vi "FipsAdjacent.vi"() -> (11 "Fips":i32[](array[numeric]))   [LabVIEW 2017] (continued)
\"Grand County, UT\"\t49019\n\"San Juan County, UT\"\t49037\t\"Kane County, UT\"\t49025\n\"San Juan County, UT\"\t49037\t\"San Juan County, UT\"\t49037\n\"San Juan County, UT\"\t49037\t\"Wayne County, UT\"\t49055\n\"Sanpete County, UT\"\t49039\t\"Carbon County, UT\"\t49007\n\"Sanpete County, UT\"\t49039\t\"Emery County, UT\"\t49015\n\"Sanpete County, UT\"\t49039\t\"Juab County, UT\"\t49023\n\"Sanpete County, UT\"\t49039\t\"Millard County, UT\"\t49027\n\"Sanpete County, UT\"\t49039\t\"Sanpete County, UT\"\t49039\n\"Sanpete County, UT\"\t49039\t\"Sevier County, UT\"\t49041\n\"Sanpete County, UT\"\t49039\t\"Utah County, UT\"\t49049\n\"Sevier County, UT\"\t49041\t\"Beaver County, UT\"\t49001\n\"Sevier County, UT\"\t49041\t\"Emery County, UT\"\t49015\n\"Sevier County, UT\"\t49041\t\"Millard County, UT\"\t49027\n\"Sevier County, UT\"\t49041\t\"Piute County, UT\"\t49031\n\"Sevier County, UT\"\t49041\t\"Sanpete County, UT\"\t49039\n\"Sevier County, UT\"\t49041\t\"Sevier County, UT\"\t49041\n\"Sevier County, UT\"\t49041\t\"Wayne County, UT\"\t49055\n\"Summit County, UT\"\t49043\t\"Daggett County, UT\"\t49009\n\"Summit County, UT\"\t49043\t\"Duchesne County, UT\"\t49013\n\"Summit County, UT\"\t49043\t\"Morgan County, UT\"\t49029\n\"Summit County, UT\"\t49043\t\"Rich County, UT\"\t49033\n\"Summit County, UT\"\t49043\t\"Salt Lake County, UT\"\t49035\n\"Summit County, UT\"\t49043\t\"Summit County, UT\"\t49043\n\"Summit County, UT\"\t49043\t\"Wasatch County, UT\"\t49051\n\"Summit County, UT\"\t49043\t\"Sweetwater County, WY\"\t56037\n\"Summit County, UT\"\t49043\t\"Uinta County, WY\"\t56041\n\"Tooele County, UT\"\t49045\t\"Elko County, NV\"\t32007\n\"Tooele County, UT\"\t49045\t\"White Pine County, NV\"\t32033\n\"Tooele County, UT\"\t49045\t\"Box Elder County, UT\"\t49003\n\"Tooele County, UT\"\t49045\t\"Davis County, UT\"\t49011\n\"Tooele County, UT\"\t49045\t\"Juab County, UT\"\t49023\n\"Tooele County, UT\"\t49045\t\"Salt Lake County, UT\"\t49035\n\"Tooele County, UT\"\t49045\t\"Tooele County, UT\"\t49045\n\"Tooele County, UT\"\t49045\t\"Utah County, UT\"\t49049\n\"Tooele County, UT\"\t49045\t\"Weber County, UT\"\t49057\n\"Uintah County, UT\"\t49047\t\"Garfield County, CO\"\t08045\n\"Uintah County, UT\"\t49047\t\"Moffat County, CO\"\t08081\n\"Uintah County, UT\"\t49047\t\"Rio Blanco County, CO\"\t08103\n\"Uintah County, UT\"\t49047\t\"Carbon County, UT\"\t49007\n\"Uintah County, UT\"\t49047\t\"Daggett County, UT\"\t49009\n\"Uintah County, UT\"\t49047\t\"Duchesne County, UT\"\t49013\n\"Uintah County, UT\"\t49047\t\"Emery County, UT\"\t49015\n\"Uintah County, UT\"\t49047\t\"Grand County, UT\"\t49019\n\"Uintah County, UT\"\t49047\t\"Uintah County, UT\"\t49047\n\"Utah County, UT\"\t49049\t\"Carbon County, UT\"\t49007\n\"Utah County, UT\"\t49049\t\"Duchesne County, UT\"\t49013\n\"Utah County, UT\"\t49049\t\"Juab County, UT\"\t49023\n\"Utah County, UT\"\t49049\t\"Salt Lake County, UT\"\t49035\n\"Utah County, UT\"\t49049\t\"Sanpete County, UT\"\t49039\n\"Utah County, UT\"\t49049\t\"Tooele County, UT\"\t49045\n\"Utah County, UT\"\t49049\t\"Utah County, UT\"\t49049\n\"Utah County, UT\"\t49049\t\"Wasatch County, UT\"\t49051\n\"Wasatch County, UT\"\t49051\t\"Duchesne County, UT\"\t49013\n\"Wasatch County, UT\"\t49051\t\"Salt Lake County, UT\"\t49035\n\"Wasatch County, UT\"\t49051\t\"Summit County, UT\"\t49043\n\"Wasatch County, UT\"\t49051\t\"Utah County, UT\"\t49049\n\"Wasatch County, UT\"\t49051\t\"Wasatch County, UT\"\t49051\n\"Washington County, UT\"\t49053\t\"Mohave County, AZ\"\t04015\n\"Washington County, UT\"\t49053\t\"Lincoln County, NV\"\t32017\n\"Washington County, UT\"\t49053\t\"Iron County, UT\"\t49021\n\"Washington County, UT\"\t49053\t\"Kane County, UT\"\t49025\n\"Washington County, UT\"\t49053\t\"Washington County, UT\"\t49053\n\"Wayne County, UT\"\t49055\t\"Emery County, UT\"\t49015\n\"Wayne County, UT\"\t49055\t\"Garfield County, UT\"\t49017\n\"Wayne County, UT\"\t49055\t\"Grand County, UT\"\t49019\n\"Wayne County, UT\"\t49055\t\"Piute County, UT\"\t49031\n\"Wayne County, UT\"\t49055\t\"San Juan County, UT\"\t49037\n\"Wayne County, UT\"\t49055\t\"Sevier County, UT\"\t49041\n\"Wayne County, UT\"\t49055\t\"Wayne County, UT\"\t49055\n\"Weber County, UT\"\t49057\t\"Box Elder County, UT\"\t49003\n\"Weber County, UT\"\t49057\t\"Cache County, UT\"\t49005\n\"Weber County, UT\"\t49057\t\"Davis County, UT\"\t49011\n\"Weber County, UT\"\t49057\t\"Morgan County, UT\"\t49029\n\"Weber County, UT\"\t49057\t\"Rich County, UT\"\t49033\n\"Weber County, UT\"\t49057\t\"Tooele County, UT\"\t49045\n\"Weber County, UT\"\t49057\t\"Weber County, UT\"\t49057\n\"Addison County, VT\"\t50001\t\"Essex County, NY\"\t36031\n\"Addison County, VT\"\t50001\t\"Washington County, NY\"\t36115\n\"Addison County, VT\"\t50001\t\"Addison County, VT\"\t50001\n\"Addison County, VT\"\t50001\t\"Chittenden County, VT\"\t50007\n\"Addison County, VT\"\t50001\t\"Orange County, VT\"\t50017\n\"Addison County, VT\"\t50001\t\"Rutland County, VT\"\t50021\n\"Addison County, VT\"\t50001\t\"Washington County, VT\"\t50023\n\"Addison County, VT\"\t50001\t\"Windsor County, VT\"\t50027\n\"Bennington County, VT\"\t50003\t\"Berkshire County, MA\"\t25003\n\"Bennington County, VT\"\t50003\t\"Franklin County, MA\"\t25011\n\"Bennington County, VT\"\t50003\t\"Rensselaer County, NY\"\t36083\n\"Bennington County, VT\"\t50003\t\"Washington County, NY\"\t36115\n\"Bennington County, VT\"\t50003\t\"Bennington County, VT\"\t50003\n\"Bennington County, VT\"\t50003\t\"Rutland County, VT\"\t50021\n\"Bennington County, VT\"\t50003\t\"Windham County, VT\"\t50025\n\"Bennington County, VT\"\t50003\t\"Windsor County, VT\"\t50027\n\"Caledonia County, VT\"\t50005\t\"Grafton County, NH\"\t33009\n\"Caledonia County, VT\"\t50005\t\"Caledonia County, VT\"\t50005\n\"Caledonia County, VT\"\t50005\t\"Essex County, VT\"\t50009\n\"Caledonia County, VT\"\t50005\t\"Lamoille County, VT\"\t50015\n\"Caledonia County, VT\"\t50005\t\"Orange County, VT\"\t50017\n\"Caledonia County, VT\"\t50005\t\"Orleans County, VT\"\t50019\n\"Caledonia County, VT\"\t50005\t\"Washington County, VT\"\t50023\n\"Chittenden County, VT\"\t50007\t\"Clinton County, NY\"\t36019\n\"Chittenden County, VT\"\t50007\t\"Essex County, NY\"\t36031\n\"Chittenden County, VT\"\t50007\t\"Addison County, VT\"\t50001\n\"Chittenden County, VT\"\t50007\t\"Chittenden County, VT\"\t50007\n\"Chittenden County, VT\"\t50007\t\"Franklin County, VT\"\t50011\n\"Chittenden County, VT\"\t50007\t\"Grand Isle County, VT\"\t50013\n\"Chittenden County, VT\"\t50007\t\"Lamoille County, VT\"\t50015\n\"Chittenden County, VT\"\t50007\t\"Washington County, VT\"\t50023\n\"Essex County, VT\"\t50009\t\"Coos County, NH\"\t33007\n\"Essex County, VT\"\t50009\t\"Grafton County, NH\"\t33009\n\"Essex County, VT\"\t50009\t\"Caledonia County, VT\"\t50005\n\"Essex County, VT\"\t50009\t\"Essex County, VT\"\t50009\n\"Essex County, VT\"\t50009\t\"Orleans County, VT\"\t50019\n\"Franklin County, VT\"\t50011\t\"Chittenden County, VT\"\t50007\n\"Franklin County, VT\"\t50011\t\"Franklin County, VT\"\t50011\n\"Franklin County, VT\"\t50011\t\"Grand Isle County, VT\"\t50013\n\"Franklin County, VT\"\t50011\t\"Lamoille County, VT\"\t50015\n\"Franklin County, VT\"\t50011\t\"Orleans County, VT\"\t50019\n\"Grand Isle County, VT\"\t50013\t\"Clinton County, NY\"\t36019\n\"Grand Isle County, VT\"\t50013\t\"Chittenden County, VT\"\t50007\n\"Grand Isle County, VT\"\t50013\t\"Franklin County, VT\"\t50011\n\"Grand Isle County, VT\"\t50013\t\"Grand Isle County, VT\"\t50013\n\"Lamoille County, VT\"\t50015\t\"Caledonia County, VT\"\t50005\n\"Lamoille County, VT\"\t50015\t\"Chittenden County, VT\"\t50007\n\"Lamoille County, VT\"\t50015\t\"Franklin County, VT\"\t50011\n\"Lamoille County, VT\"\t50015\t\"Lamoille County, VT\"\t50015\n\"Lamoille County, VT\"\t50015\t\"Orleans County, VT\"\t50019\n\"Lamoille County, VT\"\t50015\t\"Washington County, VT\"\t50023\n\"Orange County, VT\"\t50017\t\"Grafton County, NH\"\t33009\n\"Orange County, VT\"\t50017\t\"Addison County, VT\"\t50001\n\"Orange County, VT\"\t50017\t\"Caledonia County, VT\"\t50005\n\"Orange County, VT\"\t50017\t\"Orange County, VT\"\t50017\n\"Orange County, VT\"\t50017\t\"Washington County, VT\"\t50023\n\"Orange County, VT\"\t50017\t\"Windsor County, VT\"\t50027\n\"Orleans County, VT\"\t50019\t\"Caledonia County, VT\"\t50005\n\"Orleans County, VT\"\t50019\t\"Essex County, VT\"\t50009\n\"Orleans County, VT\"\t50019\t\"Franklin County, VT\"\t50011\n\"Orleans County, VT\"\t50019\t\"Lamoille County, VT\"\t50015\n\"Orleans County, VT\"\t50019\t\"Orleans County, VT\"\t50019\n\"Rutland County, VT\"\t50021\t\"Washington County, NY\"\t36115\n\"Rutland County, VT\"\t50021\t\"Addison County, VT\"\t50001\n\"Rutland County, VT\"\t50021\t\"Bennington County, VT\"\t50003\n\"Rutland County, VT\"\t50021\t\"Rutland County, VT\"\t50021\n\"Rutland County, VT\"\t50021\t\"Windsor County, VT\"\t50027\n\"Washington County, VT\"\t50023\t\"Addison County, VT\"\t50001\n\"Washington County, VT\"\t50023\t\"Caledonia County, VT\"\t50005\n\"Washington County, VT\"\t50023\t\"Chittenden County, VT\"\t50007\n\"Washington County, VT\"\t50023\t\"Lamoille County, VT\"\t50015\n\"Washington County, VT\"\t50023\t\"Orange County, VT\"\t50017\n\"Washington County, VT\"\t50023\t\"Washington County, VT\"\t50023\n\"Windham County, VT\"\t50025\t\"Franklin County, MA\"\t25011\n\"Windham County, VT\"\t50025\t\"Cheshire County, NH\"\t33005\n\"Windham County, VT\"\t50025\t\"Sullivan County, NH\"\t33019\n\"Windham County, VT\"\t50025\t\"Bennington County, VT\"\t50003\n\"Windham County, VT\"\t50025\t\"Windham County, VT\"\t50025\n\"Windham County, VT\"\t50025\t\"Windsor County, VT\"\t50027\n\"Windsor County, VT\"\t50027\t\"Grafton County, NH\"\t33009\n\"Windsor County, VT\"\t50027\t\"Sullivan County, NH\"\t33019\n\"Windsor County, VT\"\t50027\t\"Addison County, VT\"\t50001\n\"Windsor County, VT\"\t50027\t\"Bennington County, VT\"\t50003\n\"Windsor County, VT\"\t50027\t\"Orange County, VT\"\t50017\n\"Windsor County, VT\"\t50027\t\"Rutland County, VT\"\t50021\n\"Windsor County, VT\"\t50027\t\"Windham County, VT\"\t50025\n\"Windsor County, VT\"\t50027\t\"Windsor County, VT\"\t50027\n\"Accomack County, VA\"\t51001\t\"Somerset County, MD\"\t24039\n\"Accomack County, VA\"\t51001\t\"Worcester County, MD\"\t24047\n\"Accomack County, VA\"\t51001\t\"Accomack County, VA\"\t51001\n\"Accomack County, VA\"\t51001\t\"Lancaster County, VA\"\t51103\n\"Accomack County, VA\"\t51001\t\"Mathews County, VA\"\t51115\n\"Accomack County, VA\"\t51001\t\"Middlesex County, VA\"\t51119\n\"Accomack County, VA\"\t51001\t\"Northampton County, VA\"\t51131\n\"Accomack County, VA\"\t51001\t\"Northumberland County, VA\"\t51133\n\"Albemarle County, VA\"\t51003\t\"Albemarle County, VA\"\t51003\n\"Albemarle County, VA\"\t51003\t\"Augusta County, VA\"\t51015\n\"Albemarle County, VA\"\t51003\t\"Buckingham County, VA\"\t51029\n\"Albemarle County, VA\"\t51003\t\"Fluvanna County, VA\"\t51065\n\"Albemarle County, VA\"\t51003\t\"Greene County, VA\"\t51079\n\"Albemarle County, VA\"\t51003\t\"Louisa County, VA\"\t51109\n\"Albemarle County, VA\"\t51003\t\"Nelson County, VA\"\t51125\n\"Albemarle County, VA\"\t51003\t\"Orange County, VA\"\t51137\n\"Albemarle County, VA\"\t51003\t\"Rockingham County, VA\"\t51165\n\"Albemarle County, VA\"\t51003\t\"Charlottesville city, VA\"\t51540\n\"Alleghany County, VA\"\t51005\t\"Alleghany County, VA\"\t51005\n\"Alleghany County, VA\"\t51005\t\"Bath County, VA\"\t51017\n\"Alleghany County, VA\"\t51005\t\"Botetourt County, VA\"\t51023\n\"Alleghany County, VA\"\t51005\t\"Craig County, VA\"\t51045\n\"Alleghany County, VA\"\t51005\t\"Rockbridge County, VA\"\t51163\n\"Alleghany County, VA\"\t51005\t\"Covington city, VA\"\t51580\n\"Alleghany County, VA\"\t51005\t\"Greenbrier County, WV\"\t54025\n\"Alleghany County, VA\"\t51005\t\"Monroe County, WV\"\t54063\n\"Amelia County, VA\"\t51007\t\"Amelia County, VA\"\t51007\n\"Amelia County, VA\"\t51007\t\"Chesterfield County, VA\"\t51041\n\"Amelia County, VA\"\t51007\t\"Cumberland County, VA\"\t51049\n\"Amelia County, VA\"\t51007\t\"Dinwiddie County, VA\"\t51053\n\"Amelia County, VA\"\t51007\t\"Nottoway County, VA\"\t51135\n\"Amelia County, VA\"\t51007\t\"Powhatan County, VA\"\t51145\n\"Amelia County, VA\"\t51007\t\"Prince Edward County, VA\"\t51147\n\"Amherst County, VA\"\t51009\t\"Amherst County, VA\"\t51009\n\"Amherst County, VA\"\t51009\t\"Appomattox County, VA\"\t51011\n\"Amherst County, VA\"\t51009\t\"Bedford County, VA\"\t51019\n\"Amherst County, VA\"\t51009\t\"Campbell County, VA\"\t51031\n\"Amherst County, VA\"\t51009\t\"Nelson County, VA\"\t51125\n\"Amherst County, VA\"\t51009\t\"Rockbridge County, VA\"\t51163\n\"Amherst County, VA\"\t51009\t\"Lynchburg city, VA\"\t51680\n\"Appomattox County, VA\"\t51011\t\"Amherst County, VA\"\t51009\n\"Appomattox County, VA\"\t51011\t\"Appomattox County, VA\"\t51011\n\"Appomattox County, VA\"\t51011\t\"Buckingham County, VA\"\t51029\n\"Appomattox County, VA\"\t51011\t\"Campbell County, VA\"\t51031\n\"Appomattox County, VA\"\t51011\t\"Charlotte County, VA\"\t51037\n\"Appomattox County, VA\"\t51011\t\"Nelson County, VA\"\t51125\n\"Appomattox County, VA\"\t51011\t\"Prince Edward County, VA\"\t51147\n\"Arlington County, VA\"\t51013\t\"District of Columbia, DC\"\t11001\n\"Arlington County, VA\"\t51013\t\"Montgomery County, MD\"\t24031\n\"Arlington County, VA\"\t51013\t\"Arlington County, VA\"\t51013\n\"Arlington County, VA\"\t51013\t\"Fairfax County, VA\"\t51059\n\"Arlington County, VA\"\t51013\t\"Alexandria city, VA\"\t51510\n\"Arlington County, VA\"\t51013\t\"Falls Church city, VA\"\t51610\n\"Augusta County, VA\"\t51015\t\"Albemarle County, VA\"\t51003\n\"Augusta County, VA\"\t51015\t\"Augusta County, VA\"\t51015\n\"Augusta County, VA\"\t51015\t\"Bath County, VA\"\t51017\n\"Augusta County, VA\"\t51015\t\"Highland County, VA\"\t51091\n\"Augusta County, VA\"\t51015\t\"Nelson County, VA\"\t51125\n\"Augusta County, VA\"\t51015\t\"Rockbridge County, VA\"\t51163\n\"Augusta County, VA\"\t51015\t\"Rockingham County, VA\"\t51165\n\"Augusta County, VA\"\t51015\t\"Staunton city, VA\"\t51790\n\"Augusta County, VA\"\t51015\t\"Waynesboro city, VA\"\t51820\n\"Augusta County, VA\"\t51015\t\"Pendleton County, WV\"\t54071\n\"Bath County, VA\"\t51017\t\"Alleghany County, VA\"\t51005\n\"Bath County, VA\"\t51017\t\"Augusta County, VA\"\t51015\n\"Bath County, VA\"\t51017\t\"Bath County, VA\"\t51017\n\"Bath County, VA\"\t51017\t\"Highland County, VA\"\t51091\n\"Bath County, VA\"\t51017\t\"Rockbridge County, VA\"\t51163\n\"Bath County, VA\"\t51017\t\"Greenbrier County, WV\"\t54025\n\"Bath County, VA\"\t51017\t\"Pocahontas County, WV\"\t54075\n\"Bedford County, VA\"\t51019\t\"Amherst County, VA\"\t51009\n\"Bedford County, VA\"\t51019\t\"Bedford County, VA\"\t51019\n\"Bedford County, VA\"\t51019\t\"Botetourt County, VA\"\t51023\n\"Bedford County, VA\"\t51019\t\"Campbell County, VA\"\t51031\n\"Bedford County, VA\"\t51019\t\"Franklin County, VA\"\t51067\n\"Bedford County, VA\"\t51019\t\"Pittsylvania County, VA\"\t51143\n\"Bedford County, VA\"\t51019\t\"Roanoke County, VA\"\t51161\n\"Bedford County, VA\"\t51019\t\"Rockbridge County, VA\"\t51163\n\"Bedford County, VA\"\t51019\t\"Bedford city, VA\"\t51515\n\"Bedford County, VA\"\t51019\t\"Lynchburg city, VA\"\t51680\n\"Bland County, VA\"\t51021\t\"Bland County, VA\"\t51021\n\"Bland County, VA\"\t51021\t\"Giles County, VA\"\t51071\n\"Bland County, VA\"\t51021\t\"Pulaski County, VA\"\t51155\n\"Bland County, VA\"\t51021\t\"Smyth County, VA\"\t51173\n\"Bland County, VA\"\t51021\t\"Tazewell County, VA\"\t51185\n\"Bland County, VA\"\t51021\t\"Wythe County, VA\"\t51197\n\"Bland County, VA\"\t51021\t\"Mercer County, WV\"\t54055\n\"Botetourt County, VA\"\t51023\t\"Alleghany County, VA\"\t51005\n\"Botetourt County, VA\"\t51023\t\"Bedford County, VA\"\t51019\n\"Botetourt County, VA\"\t51023\t\"Botetourt County, VA\"\t51023\n\"Botetourt County, VA\"\t51023\t\"Craig County, VA\"\t51045\n\"Botetourt County, VA\"\t51023\t\"Roanoke County, VA\"\t51161\n\"Botetourt County, VA\"\t51023\t\"Rockbridge County, VA\"\t51163\n\"Brunswick County, VA\"\t51025\t\"Northampton County, NC\"\t37131\n\"Brunswick County, VA\"\t51025\t\"Warren County, NC\"\t37185\n\"Brunswick County, VA\"\t51025\t\"Brunswick County, VA\"\t51025\n\"Brunswick County, VA\"\t51025\t\"Dinwiddie County, VA\"\t51053\n\"Brunswick County, VA\"\t51025\t\"Greensville County, VA\"\t51081\n\"Brunswick County, VA\"\t51025\t\"Lunenburg County, VA\"\t51111\n\"Brunswick County, VA\"\t51025\t\"Mecklenburg County, VA\"\t51117\n\"Brunswick County, VA\"\t51025\t\"Nottoway County, VA\"\t51135\n\"Buchanan County, VA\"\t51027\t\"Pike County, KY\"\t21195\n\"Buchanan County, VA\"\t51027\t\"Buchanan County, VA\"\t51027\n\"Buchanan County, VA\"\t51027\t\"Dickenson County, VA\"\t51051\n\"Buchanan County, VA\"\t51027\t\"Russell County, VA\"\t51167\n\"Buchanan County, VA\"\t51027\t\"Tazewell County, VA\"\t51185\n\"Buchanan County, VA\"\t51027\t\"McDowell County, WV\"\t54047\n\"Buchanan County, VA\"\t51027\t\"Mingo County, WV\"\t54059\n\"Buckingham County, VA\"\t51029\t\"Albemarle County, VA\"\t51003\n\"Buckingham County, VA\"\t51029\t\"Appomattox County, VA\"\t51011\n\"Buckingham County, VA\"\t51029\t\"Buckingham County, VA\"\t51029\n\"Buckingham County, VA\"\t51029\t\"Cumberland County, VA\"\t51049\n\"Buckingham County, VA\"\t51029\t\"Fluvanna County, VA\"\t51065\n\"Buckingham County, VA\"\t51029\t\"Nelson County, VA\"\t51125\n\"Buckingham County, VA\"\t51029\t\"Prince Edward County, VA\"\t51147\n\"Campbell County, VA\"\t51031\t\"Amherst County, VA\"\t51009\n\"Campbell County, VA\"\t51031\t\"Appomattox County, VA\"\t51011\n\"Campbell County, VA\"\t51031\t\"Bedford County, VA\"\t51019\n\"Campbell County, VA\"\t51031\t\"Campbell County, VA\"\t51031\n\"Campbell County, VA\"\t51031\t\"Charlotte County, VA\"\t51037\n\"Campbell County, VA\"\t51031\t\"Halifax County, VA\"\t51083\n\"Campbell County, VA\"\t51031\t\"Pittsylvania County, VA\"\t51143\n\"Campbell County, VA\"\t51031\t\"Lynchburg city, VA\"\t51680\n\"Caroline County, VA\"\t51033\t\"Caroline County, VA\"\t51033\n\"Caroline County, VA\"\t51033\t\"Essex County, VA\"\t51057\n\"Caroline County, VA\"\t51033\t\"Hanover County, VA\"\t51085\n\"Caroline County, VA\"\t51033\t\"King and Queen County, VA\"\t51097\n\"Caroline County, VA\"\t51033\t\"King George County, VA\"\t51099\n\"Caroline County, VA\"\t51033\t\"King William County, VA\"\t51101\n\"Caroline County, VA\"\t51033\t\"Spotsylvania County, VA\"\t51177\n\"Caroline County, VA\"\t51033\t\"Stafford County, VA\"\t51179\n\"Carroll County, VA\"\t51035\t\"Surry County, NC\"\t37171\n\"Carroll County, VA\"\t51035\t\"Carroll County, VA\"\t51035\n\"Carroll County, VA\"\t51035\t\"Floyd County, VA\"\t51063\n\"Carroll County, VA\"\t51035\t\"Grayson County, VA\"\t51077\n\"Carroll County, VA\"\t51035\t\"Patrick County, VA\"\t51141\n\"Carroll County, VA\"\t51035\t\"Pulaski County, VA\"\t51155\n\"Carroll County, VA\"\t51035\t\"Wythe County, VA\"\t51197\n\"Carroll County, VA\"\t51035\t\"Galax city, VA\"\t51640\n\"Charles City County, VA\"\t51036\t\"Charles City County, VA\"\t51036\n\"Charles City County, VA\"\t51036\t\"Chesterfield County, VA\"\t51041\n\"Charles City County, VA\"\t51036\t\"Henrico County, VA\"\t51087\n\"Charles City County, VA\"\t51036\t\"James City County, VA\"\t51095\n\"Charles City County, VA\"\t51036\t\"New Kent County, VA\"\t51127\n\"Charles City County, VA\"\t51036\t\"Prince George County, VA\"\t51149\n\"Charles City County, VA\"\t51036\t\"Surry County, VA\"\t51181\n\"Charlotte County, VA\"\t51037\t\"Appomattox County, VA\"\t51011\n\"Charlotte County, VA\"\t51037\t\"Campbell County, VA\"\t51031\n\"Charlotte County, VA\"\t51037\t\"Charlotte County, VA\"\t51037\n\"Charlotte County, VA\"\t51037\t\"Halifax County, VA\"\t51083\n\"Charlotte County, VA\"\t51037\t\"Lunenburg County, VA\"\t51111\n\"Charlotte County, VA\"\t51037\t\"Mecklenburg County, VA\"\t51117\n\"Charlotte County, VA\"\t51037\t\"Prince Edward County, VA\"\t51147\n\"Chesterfield County, VA\"\t51041\t\"Amelia County, VA\"\t51007\n\"Chesterfield County, VA\"\t51041\t\"Charles City County, VA\"\t51036\n\"Chesterfield County, VA\"\t51041\t\"Chesterfield County, VA\"\t51041\n\"Chesterfield County, VA\"\t51041\t\"Dinwiddie County, VA\"\t51053\n\"Chesterfield County, VA\"\t51041\t\"Goochland County, VA\"\t51075\n\"Chesterfield County, VA\"\t51041\t\"Henrico County, VA\"\t51087\n\"Chesterfield County, VA\"\t51041\t\"Powhatan County, VA\"\t51145\n\"Chesterfield County, VA\"\t51041\t\"Prince George County, VA\"\t51149\n\"Chesterfield County, VA\"\t51041\t\"Colonial Heights city, VA\"\t51570\n\"Chesterfield County, VA\"\t51041\t\"Hopewell city, VA\"\t51670\n\"Chesterfield County, VA\"\t51041\t\"Petersburg city, VA\"\t51730\n\"Chesterfield County, VA\"\t51041\t\"Richmond city, VA\"\t51760\n\"Clarke County, VA\"\t51043\t\"Clarke County, VA\"\t51043\n\"Clarke County, VA\"\t51043\t\"Fauquier County, VA\"\t51061\n\"Clarke County, VA\"\t51043\t\"Frederick County, VA\"\t51069\n\"Clarke County, VA\"\t51043\t\"Loudoun County, VA\"\t51107\n\"Clarke County, VA\"\t51043\t\"Warren County, VA\"\t51187\n\"Clarke County, VA\"\t51043\t\"Berkeley County, WV\"\t54003\n\"Clarke County, VA\"\t51043\t\"Jefferson County, WV\"\t54037\n\"Craig County, VA\"\t51045\t\"Alleghany County, VA\"\t51005\n\"Craig County, VA\"\t51045\t\"Botetourt County, VA\"\t51023\n\"Craig County, VA\"\t51045\t\"Craig County, VA\"\t51045\n\"Craig County, VA\"\t51045\t\"Giles County, VA\"\t51071\n\"Craig County, VA\"\t51045\t\"Montgomery County, VA\"\t51121\n\"Craig County, VA\"\t51045\t\"Roanoke County, VA\"\t51161\n\"Craig County, VA\"\t51045\t\"Monroe County, WV\"\t54063\n\"Culpeper County, VA\"\t51047\t\"Culpeper County, VA\"\t51047\n\"Culpeper County, VA\"\t51047\t\"Fauquier County, VA\"\t51061\n\"Culpeper County, VA\"\t51047\t\"Madison County, VA\"\t51113\n\"Culpeper County, VA\"\t51047\t\"Orange County, VA\"\t51137\n\"Culpeper County, VA\"\t51047\t\"Rappahannock County, VA\"\t51157\n\"Culpeper County, VA\"\t51047\t\"Spotsylvania County, VA\"\t51177\n\"Culpeper County, VA\"\t51047\t\"Stafford County, VA\"\t51179\n\"Cumberland County, VA\"\t51049\t\"Amelia County, VA\"\t51007\n\"Cumberland County, VA\"\t51049\t\"Buckingham County, VA\"\t51029\n\"Cumberland County, VA\"\t51049\t\"Cumberland County, VA\"\t51049\n\"Cumberland County, VA\"\t51049\t\"Fluvanna County, VA\"\t51065\n\"Cumberland County, VA\"\t51049\t\"Goochland County, VA\"\t51075\n\"Cumberland County, VA\"\t51049\t\"Powhatan County, VA\"\t51145\n\"Cumberland County, VA\"\t51049\t\"Prince Edward County, VA\"\t51147\n\"Dickenson County, VA\"\t51051\t\"Pike County, KY\"\t21195\n\"Dickenson County, VA\"\t51051\t\"Buchanan County, VA\"\t51027\n\"Dickenson County, VA\"\t51051\t\"Dickenson County, VA\"\t51051\n\"Dickenson County, VA\"\t51051\t\"Russell County, VA\"\t51167\n\"Dickenson County, VA\"\t51051\t\"Wise County, VA\"\t51195\n\"Dinwiddie County, VA\"\t51053\t\"Amelia County, VA\"\t51007\n\"Dinwiddie County, VA\"\t51053\t\"Brunswick County, VA\"\t51025\n\"Dinwiddie County, VA\"\t51053\t\"Chesterfield County, VA\"\t51041\n\"Dinwiddie County, VA\"\t51053\t\"Dinwiddie County, VA\"\t51053\n\"Dinwiddie County, VA\"\t51053\t\"Greensville County, VA\"\t51081\n\"Dinwiddie County, VA\"\t51053\t\"Nottoway County, VA\"\t51135\n\"Dinwiddie County, VA\"\t51053\t\"Prince George County, VA\"\t51149\n\"Dinwiddie County, VA\"\t51053\t\"Sussex County, VA\"\t51183\n\"Dinwiddie County, VA\"\t51053\t\"Petersburg city, VA\"\t51730\n\"Essex County, VA\"\t51057\t\"Caroline County, VA\"\t51033\n\"Essex County, VA\"\t51057\t\"Essex County, VA\"\t51057\n\"Essex County, VA\"\t51057\t\"King and Queen County, VA\"\t51097\n\"Essex County, VA\"\t51057\t\"King George County, VA\"\t51099\n\"Essex County, VA\"\t51057\t\"Lancaster County, VA\"\t51103\n\"Essex County, VA\"\t51057\t\"Middlesex County, VA\"\t51119\n\"Essex County, VA\"\t51057\t\"Richmond County, VA\"\t51159\n\"Essex County, VA\"\t51057\t\"Westmoreland County, VA\"\t51193\n\"Fairfax County, VA\"\t51059\t\"District of Columbia, DC\"\t11001\n\"Fairfax County, VA\"\t51059\t\"Charles County, MD\"\t24017\n\"Fairfax County, VA\"\t51059\t\"Montgomery County, MD\"\t24031\n\"Fairfax County, VA\"\t51059\t\"Prince George's County, MD\"\t24033\n\"Fairfax County, VA\"\t51059\t\"Arlington County, VA\"\t51013\n\"Fairfax County, VA\"\t51059\t\"Fairfax County, VA\"\t51059\n\"Fairfax County, VA\"\t51059\t\"Loudoun County, VA\"\t51107\n\"Fairfax County, VA\"\t51059\t\"Prince William County, VA\"\t51153\n\"Fairfax County, VA\"\t51059\t\"Alexandria city, VA\"\t51510\n\"Fairfax County, VA\"\t51059\t\"Fairfax city, VA\"\t51600\n\"Fairfax County, VA\"\t51059\t\"Falls Church city, VA\"\t51610\n\"Fauquier County, VA\"\t51061\t\"Clarke County, VA\"\t51043\n\"Fauquier County, VA\"\t51061\t\"Culpeper County, VA\"\t51047\n\"Fauquier County, VA\"\t51061\t\"Fauquier County, VA\"\t51061\n\"Fauquier County, VA\"\t51061\t\"Loudoun County, VA\"\t51107\n\"Fauquier County, VA\"\t51061\t\"Prince William County, VA\"\t51153\n\"Fauquier County, VA\"\t51061\t\"Rappahannock County, VA\"\t51157\n\"Fauquier County, VA\"\t51061\t\"Stafford County, VA\"\t51179\n\"Fauquier County, VA\"\t51061\t\"Warren County, VA\"\t51187\n\"Floyd County, VA\"\t51063\t\"Carroll County, VA\"\t51035\n\"Floyd County, VA\"\t51063\t\"Floyd County, VA\"\t51063\n\"Floyd County, VA\"\t51063\t\"Franklin County, VA\"\t51067\n\"Floyd County, VA\"\t51063\t\"Montgomery County, VA\"\t51121\n\"Floyd County, VA\"\t51063\t\"Patrick County, VA\"\t51141\n\"Floyd County, VA\"\t51063\t\"Pulaski County, VA\"\t51155\n\"Floyd County, VA\"\t51063\t\"Roanoke County, VA\"\t51161\n\"Fluvanna County, VA\"\t51065\t\"Albemarle County, VA\"\t51003\n\"Fluvanna County, VA\"\t51065\t\"Buckingham County, VA\"\t51029\n\"Fluvanna County, VA\"\t51065\t\"Cumberland County, VA\"\t51049\n\"Fluvanna County, VA\"\t51065\t\"Fluvanna County, VA\"\t51065\n\"Fluvanna County, VA\"\t51065\t\"Goochland County, VA\"\t51075\n\"Fluvanna County, VA\"\t51065\t\"Louisa County, VA\"\t51109\n\"Franklin County, VA\"\t51067\t\"Bedford County, VA\"\t51019\n\"Franklin County, VA\"\t51067\t\"Floyd County, VA\"\t51063\n\"Franklin County, VA\"\t51067\t\"Franklin County, VA\"\t51067\n\"Franklin County, VA\"\t51067\t\"Henry County, VA\"\t51089\n\"Franklin County, VA\"\t51067\t\"Patrick County, VA\"\t51141\n\"Franklin County, VA\"\t51067\t\"Pittsylvania County, VA\"\t51143\n\"Franklin County, VA\"\t51067\t\"Roanoke County, VA\"\t51161\n\"Frederick County, VA\"\t51069\t\"Clarke County, VA\"\t51043\n\"Frederick County, VA\"\t51069\t\"Frederick County, VA\"\t51069\n\"Frederick County, VA\"\t51069\t\"Shenandoah County, VA\"\t51171\n\"Frederick County, VA\"\t51069\t\"Warren County, VA\"\t51187\n\"Frederick County, VA\"\t51069\t\"Winchester city, VA\"\t51840\n\"Frederick County, VA\"\t51069\t\"Berkeley County, WV\"\t54003\n\"Frederick County, VA\"\t51069\t\"Hampshire County, WV\"\t54027\n\"Frederick County, VA\"\t51069\t\"Hardy County, WV\"\t54031\n\"Frederick County, VA\"\t51069\t\"Jefferson County, WV\"\t54037\n\"Frederick County, VA\"\t51069\t\"Morgan County, WV\"\t54065\n\"Giles County, VA\"\t51071\t\"Bland County, VA\"\t51021\n\"Giles County, VA\"\t51071\t\"Craig County, VA\"\t51045\n\"Giles County, VA\"\t51071\t\"Giles County, VA\"\t51071\n\"Giles County, VA\"\t51071\t\"Montgomery County, VA\"\t51121\n\"Giles County, VA\"\t51071\t\"Pulaski County, VA\"\t51155\n\"Giles County, VA\"\t51071\t\"Mercer County, WV\"\t54055\n\"Giles County, VA\"\t51071\t\"Monroe County, WV\"\t54063\n\"Giles County, VA\"\t51071\t\"Summers County, WV\"\t54089\n\"Gloucester County, VA\"\t51073\t\"Gloucester County, VA\"\t51073\n\"Gloucester County, VA\"\t51073\t\"James City County, VA\"\t51095\n\"Gloucester County, VA\"\t51073\t\"King and Queen County, VA\"\t51097\n\"Gloucester County, VA\"\t51073\t\"Mathews County, VA\"\t51115\n\"Gloucester County, VA\"\t51073\t\"Middlesex County, VA\"\t51119\n\"Gloucester County, VA\"\t51073\t\"York County, VA\"\t51199\n\"Goochland County, VA\"\t51075\t\"Chesterfield County, VA\"\t51041\n\"Goochland County, VA\"\t51075\t\"Cumberland County, VA\"\t51049\n\"Goochland County, VA\"\t51075\t\"Fluvanna County, VA\"\t51065\n\"Goochland County, VA\"\t51075\t\"Goochland County, VA\"\t51075\n\"Goochland County, VA\"\t51075\t\"Hanover County, VA\"\t51085\n\"Goochland County, VA\"\t51075\t\"Henrico County, VA\"\t51087\n\"Goochland County, VA\"\t51075\t\"Louisa County, VA\"\t51109\n\"Goochland County, VA\"\t51075\t\"Powhatan County, VA\"\t51145\n\"Grayson County, VA\"\t51077\t\"Alleghany County, NC\"\t37005\n\"Grayson County, VA\"\t51077\t\"Ashe County, NC\"\t37009\n\"Grayson County, VA\"\t51077\t\"Surry County, NC\"\t37171\n\"Grayson County, VA\"\t51077\t\"Johnson County, TN\"\t47091\n\"Grayson County, VA\"\t51077\t\"Carroll County, VA\"\t51035\n\"Grayson County, VA\"\t51077\t\"Grayson County, VA\"\t51077\n\"Grayson County, VA\"\t51077\t\"Smyth County, VA\"\t51173\n\"Grayson County, VA\"\t51077\t\"Washington County, VA\"\t51191\n\"Grayson County, VA\"\t51077\t\"Wythe County, VA\"\t51197\n\"Grayson County, VA\"\t51077\t\"Galax city, VA\"\t51640\n\"Greene County, VA\"\t51079\t\"Albemarle County, VA\"\t51003\n\"Greene County, VA\"\t51079\t\"Greene County, VA\"\t51079\n\"Greene County, VA\"\t51079\t\"Madison County, VA\"\t51113\n\"Greene County, VA\"\t51079\t\"Orange County, VA\"\t51137\n\"Greene County, VA\"\t51079\t\"Page County, VA\"\t51139\n\"Greene County, VA\"\t51079\t\"Rockingham County, VA\"\t51165\n\"Greensville County, VA\"\t51081\t\"Northampton County, NC\"\t37131\n\"Greensville County, VA\"\t51081\t\"Brunswick County, VA\"\t51025\n\"Greensville County, VA\"\t51081\t\"Dinwiddie County, VA\"\t51053\n\"Greensville County, VA\"\t51081\t\"Greensville County, VA\"\t51081\n\"Greensville County, VA\"\t51081\t\"Southampton County, VA\"\t51175\n\"Greensville County, VA\"\t51081\t\"Sussex County, VA\"\t51183\n\"Greensville County, VA\"\t51081\t\"Emporia city, VA\"\t51595\n\"Halifax County, VA\"\t51083\t\"Caswell County, NC\"\t37033\n\"Halifax County, VA\"\t51083\t\"Granville County, NC\"\t37077\n\"Halifax County, VA\"\t51083\t\"Person County, NC\"\t37145\n\"Halifax County, VA\"\t51083\t\"Campbell County, VA\"\t51031\n\"Halifax County, VA\"\t51083\t\"Charlotte County, VA\"\t51037\n\"Halifax County, VA\"\t51083\t\"Halifax County, VA\"\t51083\n\"Halifax County, VA\"\t51083\t\"Mecklenburg County, VA\"\t51117\n\"Halifax County, VA\"\t51083\t\"Pittsylvania County, VA\"\t51143\n\"Hanover County, VA\"\t51085\t\"Caroline County, VA\"\t51033\n\"Hanover County, VA\"\t51085\t\"Goochland County, VA\"\t51075\n\"Hanover County, VA\"\t51085\t\"Hanover County, VA\"\t51085\n\"Hanover County, VA\"\t51085\t\"Henrico County, VA\"\t51087\n\"Hanover County, VA\"\t51085\t\"King William County, VA\"\t51101\n\"Hanover County, VA\"\t51085\t\"Louisa County, VA\"\t51109\n\"Hanover County, VA\"\t51085\t\"New Kent County, VA\"\t51127\n\"Hanover County, VA\"\t51085\t\"Spotsylvania County, VA\"\t51177\n\"Henrico County, VA\"\t51087\t\"Charles City County, VA\"\t51036\n\"Henrico County, VA\"\t51087\t\"Chesterfield County, VA\"\t51041\n\"Henrico County, VA\"\t51087\t\"Goochland County, VA\"\t51075\n\"Henrico County, VA\"\t51087\t\"Hanover County, VA\"\t51085\n\"Henrico County, VA\"\t51087\t\"Henrico County, VA\"\t51087\n\"Henrico County, VA\"\t51087\t\"New Kent County, VA\"\t51127\n\"Henrico County, VA\"\t51087\t\"Powhatan County, VA\"\t51145\n\"Henrico County, VA\"\t51087\t\"Richmond city, VA\"\t51760\n\"Henry County, VA\"\t51089\t\"Rockingham County, NC\"\t37157\n\"Henry County, VA\"\t51089\t\"Stokes County, NC\"\t37169\n\"Henry County, VA\"\t51089\t\"Franklin County, VA\"\t51067\n\"Henry County, VA\"\t51089\t\"Henry County, VA\"\t51089\n\"Henry County, VA\"\t51089\t\"Patrick County, VA\"\t51141\n\"Henry County, VA\"\t51089\t\"Pittsylvania County, VA\"\t51143\n\"Henry County, VA\"\t51089\t\"Martinsville city, VA\"\t51690\n\"Highland County, VA\"\t51091\t\"Augusta County, VA\"\t51015\n\"Highland County, VA\"\t51091\t\"Bath County, VA\"\t51017\n\"Highland County, VA\"\t51091\t\"Highland County, VA\"\t51091\n\"Highland County, VA\"\t51091\t\"Pendleton County, WV\"\t54071\n\"Highland County, VA\"\t51091\t\"Pocahontas County, WV\"\t54075\n\"Isle of Wight County, VA\"\t51093\t\"Isle of Wight County, VA\"\t51093\n\"Isle of Wight County, VA\"\t51093\t\"James City County, VA\"\t51095\n\"Isle of Wight County, VA\"\t51093\t\"Southampton County, VA\"\t51175\n\"Isle of Wight County, VA\"\t51093\t\"Surry County, VA\"\t51181\n\"Isle of Wight County, VA\"\t51093\t\"Franklin city, VA\"\t51620\n\"Isle of Wight County, VA\"\t51093\t\"Newport News city, VA\"\t51700\n\"Isle of Wight County, VA\"\t51093\t\"Suffolk city, VA\"\t51800\n\"James City County, VA\"\t51095\t\"Charles City County, VA\"\t51036\n\"James City County, VA\"\t51095\t\"Gloucester County, VA\"\t51073\n\"James City County, VA\"\t51095\t\"Isle of Wight County, VA\"\t51093\n\"James City County, VA\"\t51095\t\"James City County, VA\"\t51095\n\"James City County, VA\"\t51095\t\"King and Queen County, VA\"\t51097\n\"James City County, VA\"\t51095\t\"New Kent County, VA\"\t51127\n\"James City County, VA\"\t51095\t\"Surry County, VA\"\t51181\n\"James City County, VA\"\t51095\t\"York County, VA\"\t51199\n\"James City County, VA\"\t51095\t\"Newport News city, VA\"\t51700\n\"James City County, VA\"\t51095\t\"Williamsburg city, VA\"\t51830\n\"King and Queen County, VA\"\t51097\t\"Caroline County, VA\"\t51033\n\"King and Queen County, VA\"\t51097\t\"Essex County, VA\"\t51057\n\"King and Queen County, VA\"\t51097\t\"Gloucester County, VA\"\t51073\n\"King and Queen County, VA\"\t51097\t\"James City County, VA\"\t51095\n\"King and Queen County, VA\"\t51097\t\"King and Queen County, VA\"\t51097\n\"King and Queen County, VA\"\t51097\t\"King William County, VA\"\t51101\n\"King and Queen County, VA\"\t51097\t\"Middlesex County, VA\"\t51119\n\"King and Queen County, VA\"\t51097\t\"New Kent County, VA\"\t51127\n\"King George County, VA\"\t51099\t\"Charles County, MD\"\t24017\n\"King George County, VA\"\t51099\t\"Caroline County, VA\"\t51033\n\"King George County, VA\"\t51099\t\"Essex County, VA\"\t51057\n\"King George County, VA\"\t51099\t\"King George County, VA\"\t51099\n\"King George County, VA\"\t51099\t\"Stafford County, VA\"\t51179\n\"King George County, VA\"\t51099\t\"Westmoreland County, VA\"\t51193\n\"King William County, VA\"\t51101\t\"Caroline County, VA\"\t51033\n\"King William County, VA\"\t51101\t\"Hanover County, VA\"\t51085\n\"King William County, VA\"\t51101\t\"King and Queen County, VA\"\t51097\n\"King William County, VA\"\t51101\t\"King William County, VA\"\t51101\n\"King William County, VA\"\t51101\t\"New Kent County, VA\"\t51127\n\"Lancaster County, VA\"\t51103\t\"Accomack County, VA\"\t51001\n\"Lancaster County, VA\"\t51103\t\"Essex County, VA\"\t51057\n\"Lancaster County, VA\"\t51103\t\"Lancaster County, VA\"\t51103\n\"Lancaster County, VA\"\t51103\t\"Middlesex County, VA\"\t51119\n\"Lancaster County, VA\"\t51103\t\"Northumberland County, VA\"\t51133\n\"Lancaster County, VA\"\t51103\t\"Richmond County, VA\"\t51159\n\"Lee County, VA\"\t51105\t\"Bell County, KY\"\t21013\n\"Lee County, VA\"\t51105\t\"Harlan County, KY\"\t21095\n\"Lee County, VA\"\t51105\t\"Claiborne County, TN\"\t47025\n\"Lee County, VA\"\t51105\t\"Hancock County, TN\"\t47067\n\"Lee County, VA\"\t51105\t\"Lee County, VA\"\t51105\n\"Lee County, VA\"\t51105\t\"Scott County, VA\"\t51169\n\"Lee County, VA\"\t51105\t\"Wise County, VA\"\t51195\n\"Loudoun County, VA\"\t51107\t\"Frederick County, MD\"\t24021\n\"Loudoun County, VA\"\t51107\t\"Montgomery County, MD\"\t24031\n\"Loudoun County, VA\"\t51107\t\"Washington County, MD\"\t24043\n\"Loudoun County, VA\"\t51107\t\"Clarke County, VA\"\t51043\n\"Loudoun County, VA\"\t51107\t\"Fairfax County, VA\"\t51059\n\"Loudoun County, VA\"\t51107\t\"Fauquier County, VA\"\t51061\n\"Loudoun County, VA\"\t51107\t\"Loudoun County, VA\"\t51107\n\"Loudoun County, VA\"\t51107\t\"Prince William County, VA\"\t51153\n\"Loudoun County, VA\"\t51107\t\"Jefferson County, WV\"\t54037\n\"Louisa County, VA\"\t51109\t\"Albemarle County, VA\"\t51003\n\"Louisa County, VA\"\t51109\t\"Fluvanna County, VA\"\t51065\n\"Louisa County, VA\"\t51109\t\"Goochland County, VA\"\t51075\n\"Louisa County, VA\"\t51109\t\"Hanover County, VA\"\t51085\n\"Louisa County, VA\"\t51109\t\"Louisa County, VA\"\t51109\n\"Louisa County, VA\"\t51109\t\"Orange County, VA\"\t51137\n\"Louisa County, VA\"\t51109\t\"Spotsylvania County, VA\"\t51177\n\"Lunenburg County, VA\"\t51111\t\"Brunswick County, VA\"\t51025\n\"Lunenburg County, VA\"\t51111\t\"Charlotte County, VA\"\t51037\n\"Lunenburg County, VA\"\t51111\t\"Lunenburg County, VA\"\t51111\n\"Lunenburg County, VA\"\t51111\t\"Mecklenburg County, VA\"\t51117\n\"Lunenburg County, VA\"\t51111\t\"Nottoway County, VA\"\t51135\n\"Lunenburg County, VA\"\t51111\t\"Prince Edward County, VA\"\t51147\n\"Madison County, VA\"\t51113\t\"Culpeper County, VA\"\t51047\n\"Madison County, VA\"\t51113\t\"Greene County, VA\"\t51079\n\"Madison County, VA\"\t51113\t\"Madison County, VA\"\t51113\n\"Madison County, VA\"\t51113\t\"Orange County, VA\"\t51137\n\"Madison County, VA\"\t51113\t\"Page County, VA\"\t51139\n\"Madison County, VA\"\t51113\t\"Rappahannock County, VA\"\t51157\n\"Mathews County, VA\"\t51115\t\"Accomack County, VA\"\t51001\n\"Mathews County, VA\"\t51115\t\"Gloucester County, VA\"\t51073\n\"Mathews County, VA\"\t51115\t\"Mathews County, VA\"\t51115\n\"Mathews County, VA\"\t51115\t\"Middlesex County, VA\"\t51119\n\"Mathews County, VA\"\t51115\t\"Northampton County, VA\"\t51131\n\"Mathews County, VA\"\t51115\t\"York County, VA\"\t51199\n\"Mecklenburg County, VA\"\t51117\t\"Granville County, NC\"\t37077\n\"Mecklenburg County, VA\"\t51117\t\"Vance County, NC\"\t37181\n\"Mecklenburg County, VA\"\t51117\t\"Warren County, NC\"\t37185\n\"Mecklenburg County, VA\"\t51117\t\"Brunswick County, VA\"\t51025\n\"Mecklenburg County, VA\"\t51117\t\"Charlotte County, VA\"\t51037\n\"Mecklenburg County, VA\"\t51117\t\"Halifax County, VA\"\t51083\n\"Mecklenburg County, VA\"\t51117\t\"Lunenburg County, VA\"\t51111\n\"Mecklenburg County, VA\"\t51117\t\"Mecklenburg County, VA\"\t51117\n\"Middlesex County, VA\"\t51119\t\"Accomack County, VA\"\t51001\n\"Middlesex County, VA\"\t51119\t\"Essex County, VA\"\t51057\n\"Middlesex County, VA\"\t51119\t\"Gloucester County, VA\"\t51073\n\"Middlesex County, VA\"\t51119\t\"King and Queen County, VA\"\t51097\n\"Middlesex County, VA\"\t51119\t\"Lancaster County, VA\"\t51103\n\"Middlesex County, VA\"\t51119\t\"Mathews County, VA\"\t51115\n\"Middlesex County, VA\"\t51119\t\"Middlesex County, VA\"\t51119\n\"Middlesex County, VA\"\t51119\t\"Northampton County, VA\"\t51131\n\"Middlesex County, VA\"\t51119\t\"Richmond County, VA\"\t51159\n\"Montgomery County, VA\"\t51121\t\"Craig County, VA\"\t51045\n\"Montgomery County, VA\"\t51121\t\"Floyd County, VA\"\t51063\n\"Montgomery County, VA\"\t51121\t\"Giles County, VA\"\t51071\n\"Montgomery County, VA\"\t51121\t\"Montgomery County, VA\"\t51121\n\"Montgomery County, VA\"\t51121\t\"Pulaski County, VA\"\t51155\n\"Montgomery County, VA\"\t51121\t\"Roanoke County, VA\"\t51161\n\"Montgomery County, VA\"\t51121\t\"Radford city, VA\"\t51750\n\"Nelson County, VA\"\t51125\t\"Albemarle County, VA\"\t51003\n\"Nelson County, VA\"\t51125\t\"Amherst County, VA\"\t51009\n\"Nelson County, VA\"\t51125\t\"Appomattox County, VA\"\t51011\n\"Nelson County, VA\"\t51125\t\"Augusta County, VA\"\t51015\n\"Nelson County, VA\"\t51125\t\"Buckingham County, VA\"\t51029\n\"Nelson County, VA\"\t51125\t\"Nelson County, VA\"\t51125\n\"Nelson County, VA\"\t51125\t\"Rockbridge County, VA\"\t51163\n\"New Kent County, VA\"\t51127\t\"Charles City County, VA\"\t51036\n\"New Kent County, VA\"\t51127\t\"Hanover County, VA\"\t51085\n\"New Kent County, VA\"\t51127\t\"Henrico County, VA\"\t51087\n\"New Kent County, VA\"\t51127\t\"James City County, 
